vi "py-lvcomm.vi"() -> ()   [LabVIEW 2019]
uses:
  <vilib>/addons/zeromq/zmq_context.lvclass
  <vilib>/addons/zeromq/zmq_socket.lvclass
  <userlib>/LevyLab/Transport/Control Experiment/Control Experiment.lvclass
  <vilib>/addons/zeromq/socket_type.ctl
  <userlib>/LevyLab/Instrument Framework/Instrument Types/Cryostat/Instrument.Cryostat.lvclass
  <vilib>/addons/zeromq/zeromq.lvlib
  <userlib>/LevyLab/Lockin-Multichannel/Instrument.Lockin/Instrument.Lockin.lvclass
panel:
  out "Status":string
  out "Command":string
  in  "Exit":bool
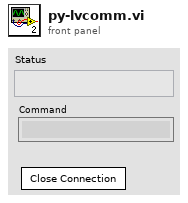
[diagram p1: front panel]
types:
  T1 = enum32{"Invalid", "Standard", "Closed", "Hidden", "Minimized", "Maximized"}
  T2 = enum32{"invalid app kind", "Development System", "Run Time System", "Student Edition", "Embedded LabVIEW", "Evaluation", "Custom"}
  T3 = typedef "zeromq.lvlib/socket_type.ctl" = enum8{"ZMQ_PAIR", "ZMQ_PUB", "ZMQ_SUB", "ZMQ_REQ", "ZMQ_REP", "ZMQ_DEALER", "ZMQ_ROUTER", "ZMQ_PULL", "ZMQ_PUSH", "ZMQ_XPUB", "ZMQ_XSUB", "ZMQ_STREAM", "ZMQ_SERVER", "ZMQ_CLIENT", "ZMQ_RADIO", "ZMQ_DISH", "ZMQ_GATHER", "ZMQ_SCATTER", "ZMQ_DGRAM"}
  T4 = cluster{"Core":cluster{"Current VI Reference":refnum<vi>, "Close Panel on Exit?":bool}, "ZMQ":cluster{"Context":refnum<class "zmq_context.lvclass">, "Socket":refnum<class "zmq_socket.lvclass">}, "C.E.":refnum<class "Control Experiment.lvclass">, "Command":cluster{"Command":string, "Args":string}}
  T5 = cluster{"Context":refnum<class "zmq_context.lvclass">, "Socket":refnum<class "zmq_socket.lvclass">}
  T6 = cluster{"Current VI Reference":refnum<vi>, "Close Panel on Exit?":bool}
  T7 = typedef "Control Experiment.lvclass/Instrument Classes--cluster.ctl" = cluster{"KH7008":refnum<class "Instrument.KH7008.lvclass">[], "Lockin":refnum<class "Instrument.Lockin.lvclass">, "Temperature":refnum<class "Instrument.Cryostat.lvclass">, "Magnet":refnum<class "Instrument.Cryostat.lvclass">, "Rotator":refnum<class "Instrument.Cryostat.lvclass">, "Level":refnum<class "Instrument.Cryostat.lvclass">, "Capacitance Bridge":refnum<class "Instrument.CBridge.lvclass">, "Delay Line":refnum<class "Instrument.DelayLine.lvclass">, "Strain Cell":refnum<class "Instrument.Strain.lvclass">, "VNA":refnum<class "Instrument.VNA.lvclass">, "Voltage Source":refnum<class "Instrument.VSource.lvclass">}
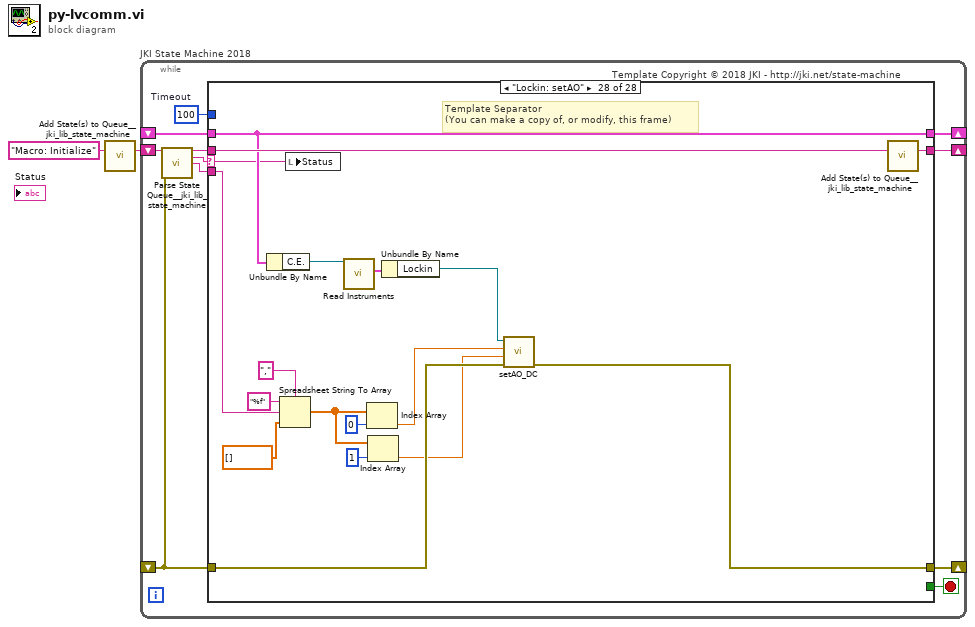
[diagram p0: block diagram]
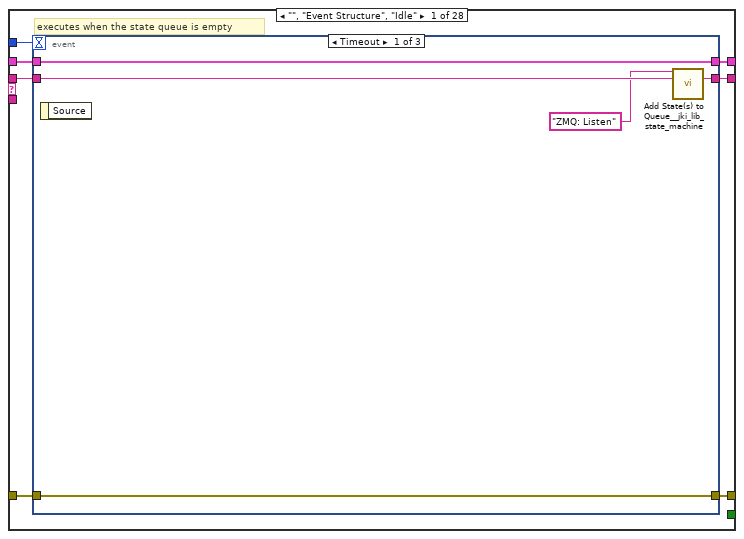
[diagram p2: hidden frame]
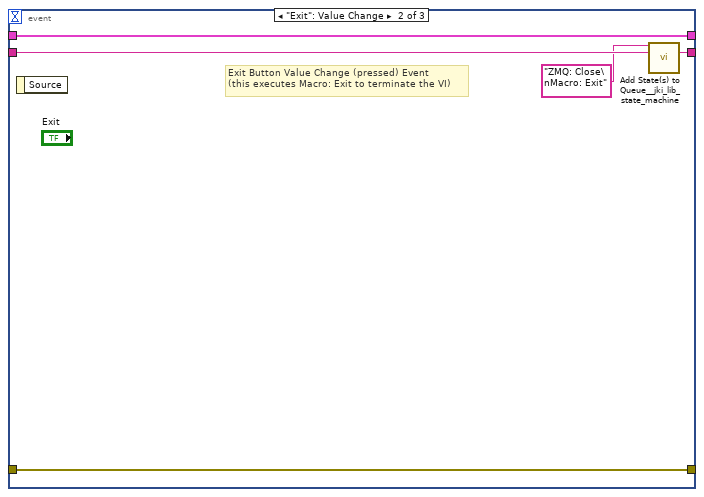
[diagram p3: hidden frame]
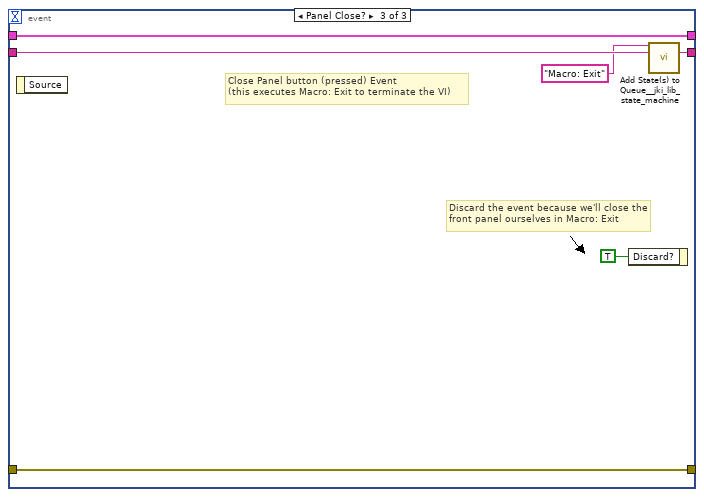
[diagram p4: hidden frame]
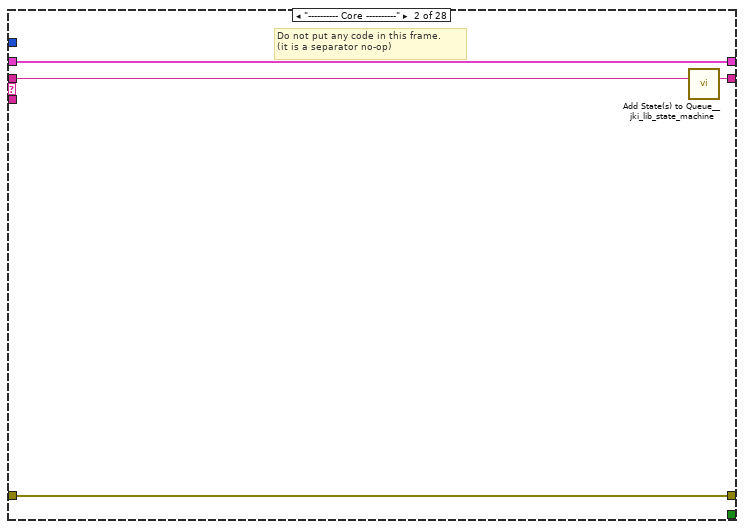
[diagram p5: hidden frame]
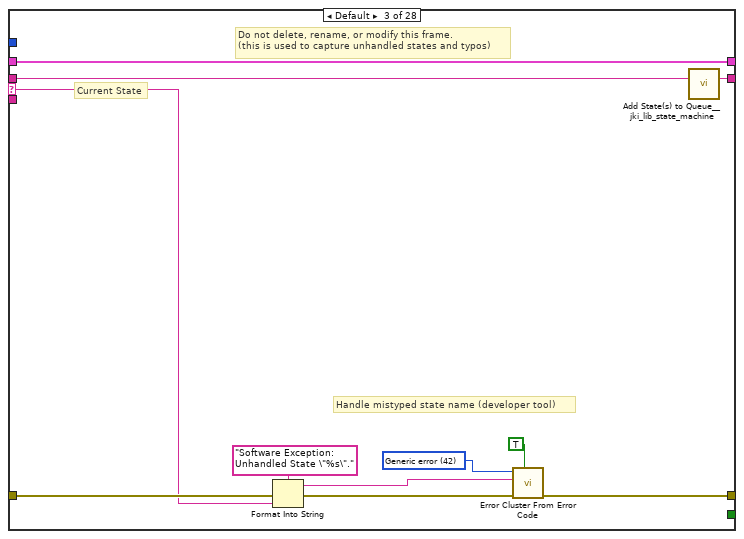
[diagram p6: hidden frame]
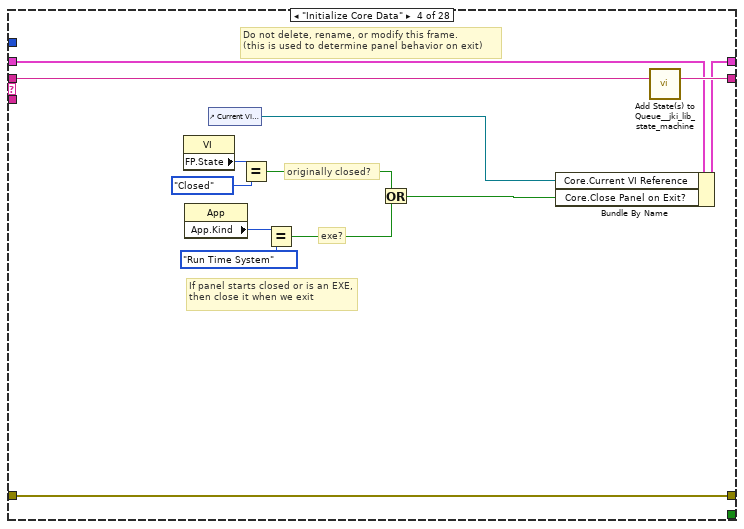
[diagram p7: hidden frame]
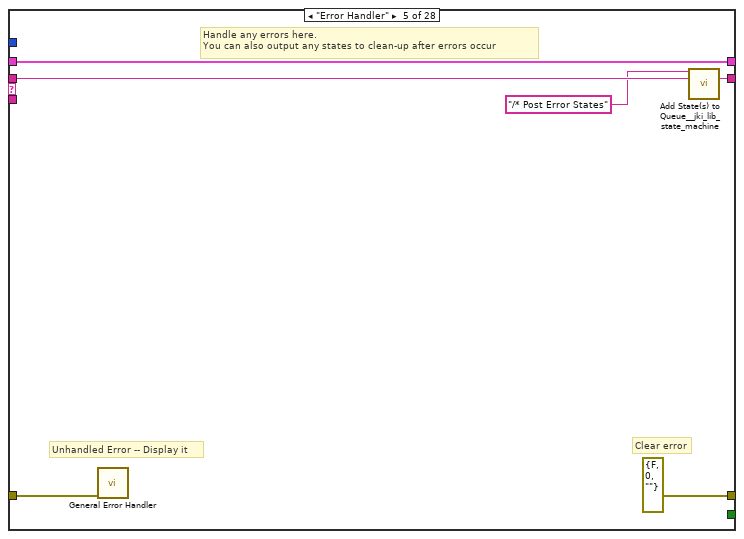
[diagram p8: hidden frame]
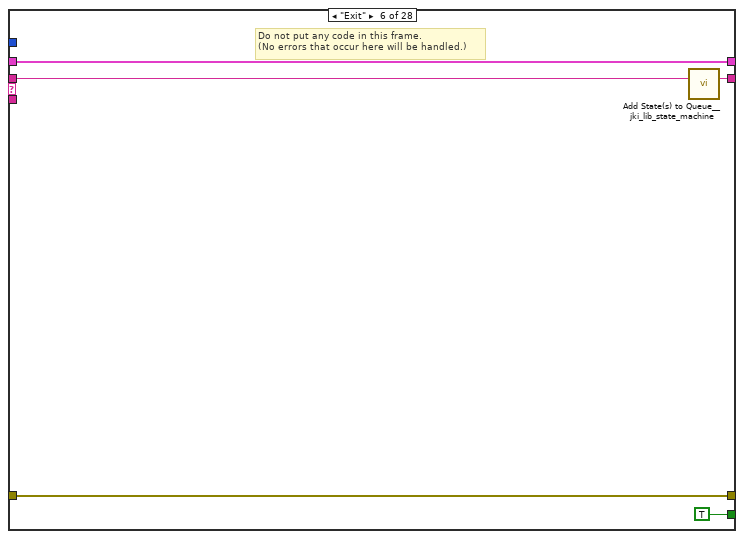
[diagram p9: hidden frame]
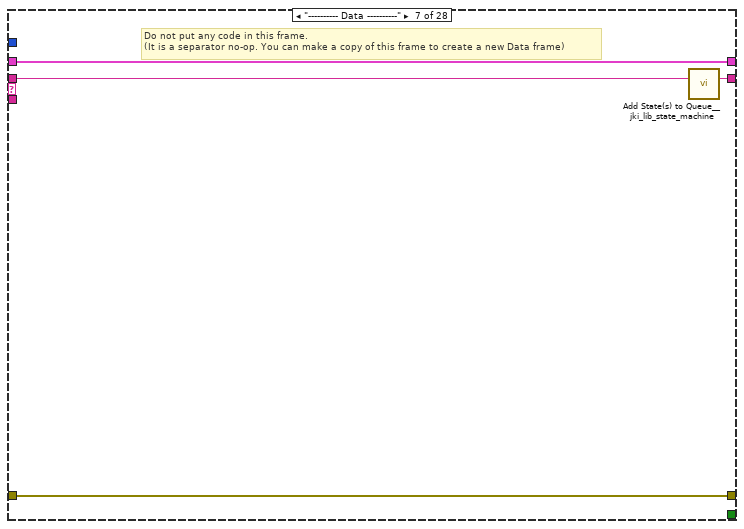
[diagram p10: hidden frame]
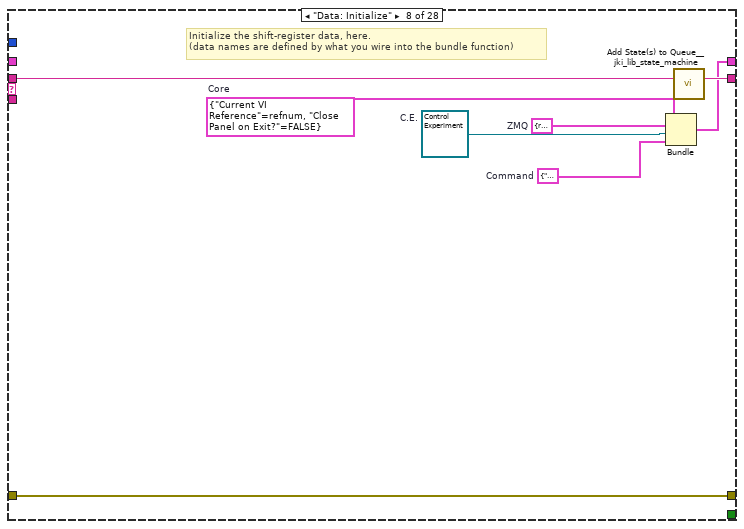
[diagram p11: hidden frame]
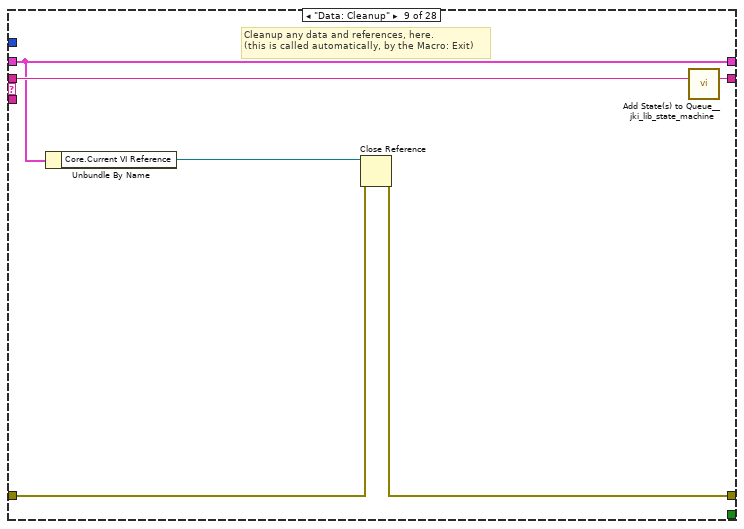
[diagram p12: hidden frame]
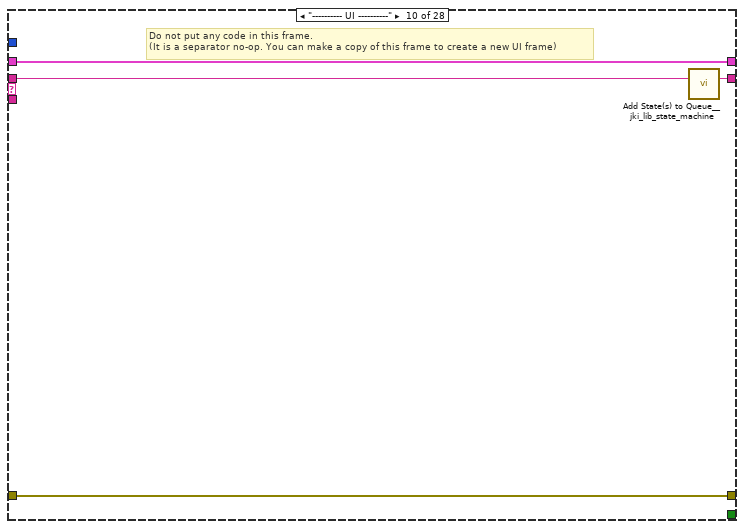
[diagram p13: hidden frame]
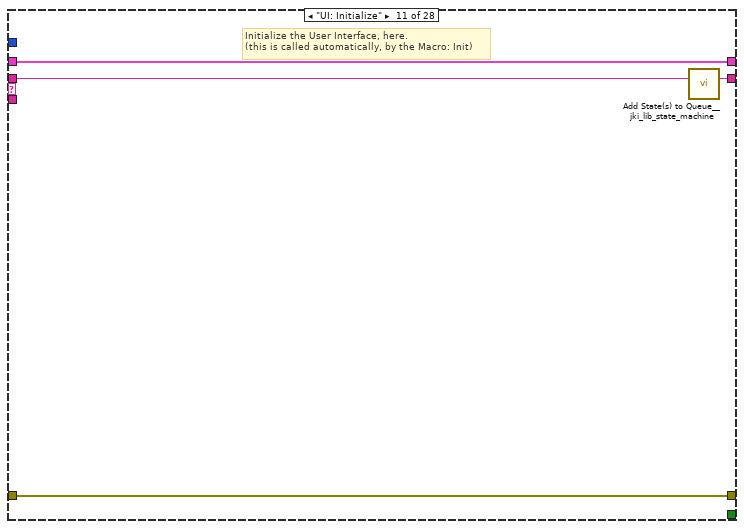
[diagram p14: hidden frame]
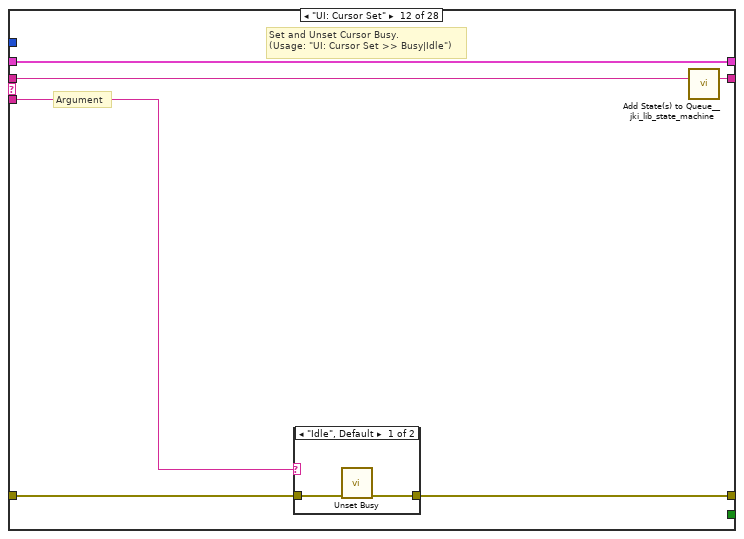
[diagram p15: hidden frame]
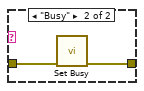
[diagram p16: hidden frame]
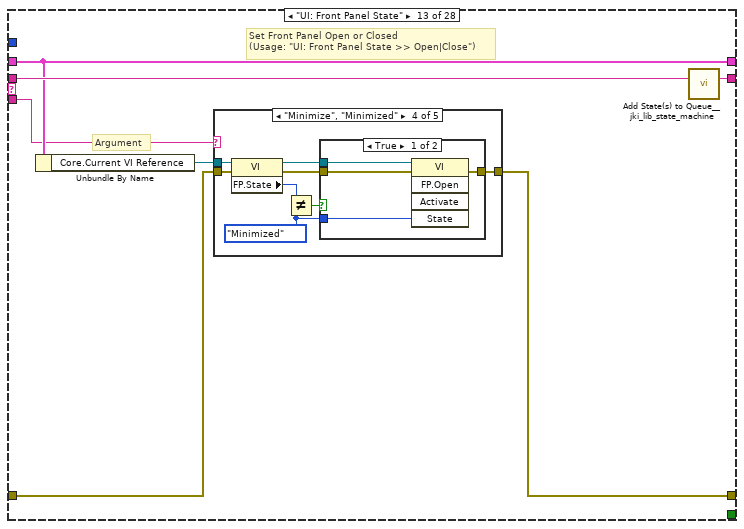
[diagram p17: hidden frame]
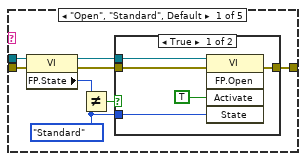
[diagram p18: hidden frame]
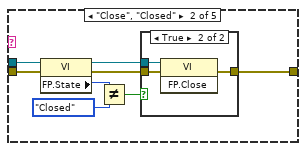
[diagram p20: hidden frame]
diagram:
  n1 = call <vilib>:"Add State(s) to Queue__jki_lib_state_machine.vi"("State(s) in (\"\")"="Macro: Initialize") -> ("States Out"=w2:string)  [unwired: 14 in]
  n2 = while "JKI State Machine 2018" {
    shift-right: [w6] -> _
    shift-left: _ -> [w5]
    shift-right: [w9] -> _
    shift-left: _ -> [w3]
    shift-right: [w8] -> _
    shift-left: w2 -> [w10]
    stop <- w7 stop-if-true
    w4 = 100  # Timeout
    # "Template Copyright © 2018 JKI - http://jki.net/state-machine"
    n3 = call <vilib>:"Parse State Queue__jki_lib_state_machine.vi"("State Queue"=w10, "Error In (no error)"=w3) -> ("Remaining States"=w12:string, "Current State"=w13:string, "Arguments"=w11:string)  [unwired: 11 in]
    n4 = case shown="\"Lockin: setAO\"" w13 {
      selector: w13 -> [_ _ w41 _ _ _ _ _ _ _ _ _ _ _ _ _ _ w207 w228 w245 _ _ _ _ w292 w311 _ w334]
      tunnel: w12 -> [w20 w40 w45 w64 w70 w75 w79 w87 w93 w97 w101 w107 w118 w187 w192 w202 w206 w221 w242 w250 w266 w270 w278 w282 w301 w320 w324 w342]
      tunnel: w11 -> [_ _ _ _ _ _ _ _ _ _ _ w102 w112 _ _ _ _ _ _ _ _ _ _ _ w291 w310 _ w327]
      tunnel: w5 -> [w18 w37 w43 w57 w67 w73 w76 _ w88 w94 w99 w105 w114 w184 w189 w199 w203 w211 w236 w246 w264 w267 w275 w279 w298 w317 w321 w338]
      tunnel: [w17 w38 w47 w61 errorcluster {"status"=FALSE, "code"=0, "source"=""} ("error out") w72 w77 w84 w89 w95 w98 w103 w115 w185 w190 w200 w204 w212 w233 w247 w259 w268 w273 w280 w294 w313 w322 w339] -> w9
      tunnel: w3 -> [w16 w38 w46 w61 w66 w72 w77 w84 w90 w95 w98 w104 w116 w185 w190 w200 w204 w216 w239 w247 w261 w268 w272 w280 w296 w315 w322 w340]
      tunnel: [w19 w39 w44 w63 w69 w74 w78 w86 w92 w96 w100 w106 w117 w186 w191 w201 w205 w220 w241 w249 w265 w269 w277 w281 w300 w319 w323 w341] -> w8
      tunnel: [_ _ _ _ _ TRUE _ _ _ _ _ _ _ _ _ _ _ _ _ _ _ _ _ _ _ _ _ _] -> w7
      tunnel: [w15 w37 w43 w62 w67 w73 w76 w85 w88 w94 w99 w105 w114 w184 w189 w199 w203 w210 w235 w246 w264 w267 w271 w279 w298 w317 w321 w338] -> w6
      tunnel: w4 -> [w14 _ _ _ _ _ _ _ _ _ _ _ _ _ _ _ _ _ _ _ _ _ _ _ _ _ _ _]
      frame "", "Event Structure", "Idle" {
        # "executes when the state queue is empty"
        n5 = event shown="[0] Timeout" {
          selector: _ -> [_ _ _]
          dyn-events: _ -> [_ _ _]
          timeout: w14 -> [_ _ _]
          tunnel: w20 -> [w25 w30 w36]
          tunnel: [w24 w29 w35] -> w19
          tunnel: w18 -> [w22 w27 w33]
          tunnel: [w23 w28 w34] -> w17
          tunnel: w16 -> [w23 w28 w34]
          tunnel: [w22 w27 w33] -> w15
          event Timeout {
            n6 = event-data() -> ()  [unwired: 1 in, 1 out]
            n7 = call <vilib>:"Add State(s) to Queue__jki_lib_state_machine.vi"("State(s) in Front (\"\")"="ZMQ: Listen" ("State(s) in Front (\"\")"), "State(s) in (\"\")"=w25) -> ("States Out"=w24:string)  [unwired: 13 in]
          }
          event "Exit": Value Change {
            # "Exit Button Value Change (pressed) Event\n(this executes Macro: Exit to terminate the VI)"
            n8 = event-data() -> ()  [unwired: 1 in, 1 out]
            n9 = call <vilib>:"Add State(s) to Queue__jki_lib_state_machine.vi"("State(s) in Front (\"\")"="ZMQ: Close\nMacro: Exit", "State(s) in (\"\")"=w30) -> ("States Out"=w29:string)  [unwired: 13 in]
          }
          event Panel Close? {
            # "Discard the event because we'll close the front panel ourselves in Macro: Exit"
            # "Close Panel button (pressed) Event\n(this executes Macro: Exit to terminate the VI)"
            n10 = event-data() -> ()  [unwired: 1 in, 1 out]
            n11 = event-data("Discard?"=TRUE) -> ()  [unwired: 1 in, 1 out]
            n12 = call <vilib>:"Add State(s) to Queue__jki_lib_state_machine.vi"("State(s) in Front (\"\")"="Macro: Exit", "State(s) in (\"\")"=w36) -> ("States Out"=w35:string)  [unwired: 13 in]
          }
        }
      }
      frame "---------- Core ----------" {
        # "Do not put any code in this frame.\n(it is a separator no-op)"
        n13 = call <vilib>:"Add State(s) to Queue__jki_lib_state_machine.vi"("State(s) in (\"\")"=w40) -> ("States Out"=w39:string)  [unwired: 14 in]
      }
      frame Default {
        w50 = 42 items=["No error", "Argument error", "Memory is full", "Out of zone", "End of file", "File already open", "Generic file I/O error", "File not found", "File permission error", "Disk is full", "Duplicate path", "Too many files open", "System feature not enabled", "Resource file not found", "Cannot add resource", "Resource not found", "Image not found", "Image memory error", "Pen does not exist", "Config type invalid", "Config token not found", "Config parse error", "Config memory error", "Bad external code format", "Bad external code offset", "External code not present", "Null window", "Destroy window error", "Null menu", "Print aborted", "Bad print record", "Print driver error", "Windows error during printing", "Memory error during printing", "Print dialog error", "Generic print error", "Invalid device refnum", "Device not found", "Device parameter error", "Device unit error", "Cannot open device", "Device call aborted", "Generic error", "Cancelled by user", "Object ID too low", "Object ID too high", "Object not in heap", "Unknown heap", "Unknown object (invalid DefProc)", "Unknown object (DefProc not in table)", "Message out of range", "Invalid (null) method", "Unknown message", "Manager call not supported", "Bad address", "Network operation in progress", "Network operation timed out", "Connection is busy", "Network attribute not supported", "Network error", "Address in use", "System out of memory", "Connection aborted", "Connection refused", "Not connected", "Already connected", "Connection closed", "Initialization error (interapplication manager)", "Bad occurrence", "Wait on unbound occurrence handler", "Occurrence queue overflow", "Datalog type conflict", "Unused", "Unrecognized type (interapplication manager)", "Memory corrupt", "Failed to make temporary DLL", "Old CIN version", "Drag socket not found", "Failed to load drop-object", "Failed to register OLE object", "Failed to release OLE object", "Format specifier type mismatch", "Unknown format specifier", "Too few format specifiers", "Too many format specifiers", "Scan failed", "Newer CIN version", "Error converting to variant", "Runtime menu error", "Password tampered", "Variant attribute not found", "Incompatible variant data type", "Event data is not available", "Event Store is not present", "Occurrence is not found", "Event Queue is not created", "Event info is not available", "Refnum passed is NULL", "Error retrieving Class GUID", "Error retrieving CoClass GUID", "Error retrieving TypeLib GUID.", "Bad built application magic bytes.", "Specific driver is different from the specific driver associated with the Logical Name.", "There is no session opened to the class driver.", "Max Error", "MAX - Error with config objects", "MAX - Error loading configuration", "MAX - Group not supported"]
        # "Current State"
        # "Do not delete, rename, or modify this frame.\n(this is used to capture unhandled states and typos)"
        # "Handle mistyped state name (developer tool)"
        n14 = Format Into String(format string="Software Exception: Unhandled State \"%s\"." ("message"), error in=w46, w41) -> (resulting string=w49:string, error out=w48:errorcluster)  [unwired: 1 in]
        n15 = call <vilib>:"Error Cluster From Error Code.vi"("show call chain? (False)"=TRUE, "error in (no error)"=w48, "error message (\"\")"=w49, "error code (0)"=w50) -> ("error out"=w47:errorcluster)  [unwired: 5 in]
        n16 = call <vilib>:"Add State(s) to Queue__jki_lib_state_machine.vi"("State(s) in (\"\")"=w45) -> ("States Out"=w44:string)  [unwired: 14 in]
      }
      frame "Initialize Core Data" {
        # "Do not delete, rename, or modify this frame.\n(this is used to determine panel behavior on exit)"
        # "originally closed?"
        # "exe?"
        # "If panel starts closed or is an EXE, then close it when we exit"
        n17 = property class="VI"() -> ("FP.State"=w54:T1)  [unwired: 2 in, 2 out]
        n18 = property class="App"() -> ("App.Kind"=w60:T2)  [unwired: 2 in, 2 out]
        n19 = control-ref of="Current VI Reference"() -> (w55:refnum<vi>)
        n20 = Equal?(x=w54, y=T1."Closed" ("Front Panel Window:State")) -> (x = y?=w52:bool)
        n21 = Equal?(x=w60, y=T2."Run Time System" ("Application:Kind")) -> (x = y?=w58:bool)
        n22 = Or(x=w52, y=w58) -> (x .or. y?=w56:bool)
        n23 = Bundle By Name(cluster=w57, "Core.Current VI Reference"=w55, "Core.Close Panel on Exit?"=w56) -> (w62:T4)
        n24 = call <vilib>:"Add State(s) to Queue__jki_lib_state_machine.vi"("State(s) in (\"\")"=w64) -> ("States Out"=w63:string)  [unwired: 14 in]
      }
      frame "Error Handler" {
        # "Unhandled Error -- Display it"
        # "Handle any errors here.\nYou can also output any states to clean-up after errors occur"
        # "Clear error"
        n25 = call <vilib>:"General Error Handler.vi"("error in (no error)"=w66) -> ()  [unwired: 10 in, 5 out]
        n26 = call <vilib>:"Add State(s) to Queue__jki_lib_state_machine.vi"("State(s) in Front (\"\")"="/* Post Error States", "State(s) in (\"\")"=w70) -> ("States Out"=w69:string)  [unwired: 13 in]
      }
      frame "Exit" {
        # "Do not put any code in this frame.\n(No errors that occur here will be handled.)"
        n27 = call <vilib>:"Add State(s) to Queue__jki_lib_state_machine.vi"("State(s) in (\"\")"=w75) -> ("States Out"=w74:string)  [unwired: 14 in]
      }
      frame "---------- Data ----------" {
        # "Do not put any code in this frame.\n(It is a separator no-op. You can make a copy of this frame to create a new Data frame)"
        n28 = call <vilib>:"Add State(s) to Queue__jki_lib_state_machine.vi"("State(s) in (\"\")"=w79) -> ("States Out"=w78:string)  [unwired: 14 in]
      }
      frame "Data: Initialize" {
        w80 = cluster{"Command":string, "Args":string} {"Command"="", "Args"=""}  # Command
        w81 = refnum<class "Control Experiment.lvclass"> refnum  # C.E.
        w82 = T5 {"Context"=refnum, "Socket"=refnum}  # ZMQ
        w83 = T6 {"Current VI Reference"=refnum, "Close Panel on Exit?"=FALSE}  # Core
        # "Initialize the shift-register data, here.\n(data names are defined by what you wire into the bundle function)"
        n29 = Bundle("Core"=w83, "ZMQ"=w82, "C.E."=w81, "Command"=w80) -> (w85:T4)  [unwired: 1 in]
        n30 = call <vilib>:"Add State(s) to Queue__jki_lib_state_machine.vi"("State(s) in (\"\")"=w87) -> ("States Out"=w86:string)  [unwired: 14 in]
      }
      frame "Data: Cleanup" {
        # "Cleanup any data and references, here.\n(this is called automatically, by the Macro: Exit)"
        n31 = Unbundle By Name(w88) -> ("Core.Current VI Reference"=w91:refnum<vi>)
        n32 = Close Reference(reference=w91, error in (no error)=w90) -> (error out=w89:errorcluster)
        n33 = call <vilib>:"Add State(s) to Queue__jki_lib_state_machine.vi"("State(s) in (\"\")"=w93) -> ("States Out"=w92:string)  [unwired: 14 in]
      }
      frame "---------- UI ----------" {
        # "Do not put any code in this frame.\n(It is a separator no-op. You can make a copy of this frame to create a new UI frame)"
        n34 = call <vilib>:"Add State(s) to Queue__jki_lib_state_machine.vi"("State(s) in (\"\")"=w97) -> ("States Out"=w96:string)  [unwired: 14 in]
      }
      frame "UI: Initialize" {
        # "Initialize the User Interface, here.\n(this is called automatically, by the Macro: Init)"
        n35 = call <vilib>:"Add State(s) to Queue__jki_lib_state_machine.vi"("State(s) in (\"\")"=w101) -> ("States Out"=w100:string)  [unwired: 14 in]
      }
      frame "UI: Cursor Set" {
        # "Argument"
        # "Set and Unset Cursor Busy.\n(Usage: \"UI: Cursor Set >> Busy|Idle\")"
        n36 = case shown="\"Idle\", Default" w102 {
          tunnel: w104 -> [w109 w111]
          tunnel: [w108 w110] -> w103
          frame "Idle", Default {
            n37 = call <vilib>:"Unset Busy.vi"("error in (no error)"=w109) -> ("error out"=w108:errorcluster)  [unwired: 10 in]
          }
          frame "Busy" {
            n38 = call <vilib>:"Set Busy.vi"("error in (no error)"=w111) -> ("error out"=w110:errorcluster)  [unwired: 9 in, 1 out]
          }
        }
        n39 = call <vilib>:"Add State(s) to Queue__jki_lib_state_machine.vi"("State(s) in (\"\")"=w107) -> ("States Out"=w106:string)  [unwired: 14 in]
      }
      frame "UI: Front Panel State" {
        # "Argument"
        # "Set Front Panel Open or Closed\n(Usage: \"UI: Front Panel State >> Open|Close\")"
        n40 = Unbundle By Name(w114) -> ("Core.Current VI Reference"=w113:refnum<vi>)
        n41 = case shown="\"Minimize\", \"Minimized\"" w112 {
          tunnel: w116 -> [w124 w139 w150 w163 w176]
          tunnel: [w126 w140 w152 w165 w178] -> w115
          tunnel: w113 -> [w125 w137 w151 w164 w177]
          frame "Open", "Standard", Default {
            w119 = T1."Standard" ("State")
            n42 = property class="VI"(reference=w125, error in=w124) -> (reference out=w122:refnum<vi>, error out=w123:errorcluster, "FP.State"=w121:T1)
            n43 = Not Equal?(x=w121, y=w119) -> (x != y?=w120:bool)
            n44 = case shown="True" w120 {
              tunnel: [w130 w132] -> w126
              tunnel: w123 -> [w129 w132]
              tunnel: w122 -> [w128 _]
              tunnel: w119 -> [w127 _]
              frame True {
                n45 = invoke class="VI" method="FP.Open"(reference=w128, error in=w129, "Activate"=TRUE, "State"=w127) -> (error out=w130:errorcluster)  [unwired: 1 in, 4 out]
              }
              frame False {
              }
            }
          }
          frame "Close", "Closed" {
            n46 = property class="VI"(reference=w137, error in=w139) -> (reference out=w136:refnum<vi>, error out=w138:errorcluster, "FP.State"=w134:T1)
            n47 = Not Equal?(x=w134, y=T1."Closed" ("Front Panel Window:State")) -> (x != y?=w133:bool)
            n48 = case shown="True" w133 {
              tunnel: [w141 w144] -> w140
              tunnel: w138 -> [w141 w143]
              tunnel: w136 -> [_ w142]
              frame False {
              }
              frame True {
                n49 = invoke class="VI" method="FP.Close"(reference=w142, error in=w143) -> (error out=w144:errorcluster)  [unwired: 1 in, 2 out]
              }
            }
          }
          frame "Hidden", "Hide" {
            w145 = T1."Hidden" ("State")
            n50 = property class="VI"(reference=w151, error in=w150) -> (reference out=w148:refnum<vi>, error out=w149:errorcluster, "FP.State"=w147:T1)
            n51 = Not Equal?(x=w147, y=w145) -> (x != y?=w146:bool)
            n52 = case shown="True" w146 {
              tunnel: [w156 w157] -> w152
              tunnel: w149 -> [w155 w157]
              tunnel: w148 -> [w154 _]
              tunnel: w145 -> [w153 _]
              frame True {
                n53 = invoke class="VI" method="FP.Open"(reference=w154, error in=w155, "State"=w153) -> (error out=w156:errorcluster)  [unwired: 2 in, 4 out]
              }
              frame False {
              }
            }
          }
          frame "Minimize", "Minimized" {
            w158 = T1."Minimized" ("State")
            n54 = property class="VI"(reference=w164, error in=w163) -> (reference out=w161:refnum<vi>, error out=w162:errorcluster, "FP.State"=w160:T1)
            n55 = Not Equal?(x=w160, y=w158) -> (x != y?=w159:bool)
            n56 = case shown="True" w159 {
              tunnel: [w169 w170] -> w165
              tunnel: w162 -> [w168 w170]
              tunnel: w161 -> [w167 _]
              tunnel: w158 -> [w166 _]
              frame True {
                n57 = invoke class="VI" method="FP.Open"(reference=w167, error in=w168, "State"=w166) -> (error out=w169:errorcluster)  [unwired: 2 in, 4 out]
              }
              frame False {
              }
            }
          }
          frame "Maximize", "Maximized" {
            w171 = T1."Maximized" ("State")
            n58 = property class="VI"(reference=w177, error in=w176) -> (reference out=w174:refnum<vi>, error out=w175:errorcluster, "FP.State"=w173:T1)
            n59 = Not Equal?(x=w173, y=w171) -> (x != y?=w172:bool)
            n60 = case shown="True" w172 {
              tunnel: [w182 w183] -> w178
              tunnel: w175 -> [w181 w183]
              tunnel: w174 -> [w180 _]
              tunnel: w171 -> [w179 _]
              frame True {
                n61 = invoke class="VI" method="FP.Open"(reference=w180, error in=w181, "State"=w179) -> (error out=w182:errorcluster)  [unwired: 2 in, 4 out]
              }
              frame False {
              }
            }
          }
        }
        n62 = call <vilib>:"Add State(s) to Queue__jki_lib_state_machine.vi"("State(s) in (\"\")"=w118) -> ("States Out"=w117:string)  [unwired: 14 in]
      }
      frame "---------- Macro ----------" {
        # "Do not put any code in this frame.\n(It is a separator no-op. You can make a copy of this frame to create a new Macro frame)"
        n63 = call <vilib>:"Add State(s) to Queue__jki_lib_state_machine.vi"("State(s) in (\"\")"=w187) -> ("States Out"=w186:string)  [unwired: 14 in]
      }
      frame "Macro: Initialize" {
        w188 = "Data: Initialize\nInitialize Core Data\nUI: Initialize\nUI: Front Panel State >> Open\nCE: Init\nZMQ: Init"  # Data: Initialize Initialize Core Data UI: Initialize UI: Front Panel State >> Open CE: Init ZMQ: Init
        # "Initialization Macro\n(This is called once, when the VI starts)"
        n64 = call <vilib>:"Add State(s) to Queue__jki_lib_state_machine.vi"("State(s) in Front (\"\")"=w188, "State(s) in (\"\")"=w192) -> ("States Out"=w191:string)  [unwired: 13 in]
      }
      frame "Macro: Exit" {
        # "Exit Macro\n(This is called once, when the VI exits)"
        n65 = Unbundle By Name(w199) -> ("Core.Close Panel on Exit?"=w198:bool)
        n66 = Select(t="UI: Front Panel State >> Close", s=w198, f="") -> (s? t:f=w195:string)
        n67 = call <vilib>:"Add State(s) to Queue__jki_lib_state_machine.vi"("State(s) in (\"\")"=w195, "State(s) at Back (\"\")"="Data: Cleanup\nExit") -> ("States Out"=w193:string)  [unwired: 13 in]
        n68 = call <vilib>:"Add State(s) to Queue__jki_lib_state_machine.vi"("State(s) in Front (\"\")"=w193, "State(s) in (\"\")"=w202) -> ("States Out"=w201:string)  [unwired: 13 in]
      }
      frame "---------- ZMQ ----------" {
        # "Template Separator\n(You can make a copy of, or modify, this frame)"
        n69 = call <vilib>:"Add State(s) to Queue__jki_lib_state_machine.vi"("State(s) in (\"\")"=w206) -> ("States Out"=w205:string)  [unwired: 14 in]
      }
      frame "ZMQ: Init" {
        n70 = local write "Status"(w207) -> ()
        n71 = call <vilib>:"zmq_ctx_create.vi"("error in"=w216) -> ("error out"=w215:errorcluster, "context out"=w219:refnum<class "zmq_context.lvclass">)  [unwired: 3 in]
        n72 = call <vilib>:"zmq_socket.vi"("error in"=w215, "socket type"=socket_type."ZMQ_REP", "context in"=w219) -> ("error out"=w213:errorcluster, "socket out"=w217:refnum<class "zmq_socket.lvclass">, "context out"=w209:refnum<class "zmq_context.lvclass">)  [unwired: 2 in]
        n73 = call <vilib>:"zmq_bind.vi"("error in"=w213, "endpoint"="tcp://*:15555", "socket in"=w217) -> ("error out"=w212:errorcluster, "socket out"=w208:refnum<class "zmq_socket.lvclass">)  [unwired: 1 in]
        n74 = Bundle By Name(cluster=w211, "ZMQ.Context"=w209, "ZMQ.Socket"=w208) -> (w210:T4)
        n75 = call <vilib>:"Add State(s) to Queue__jki_lib_state_machine.vi"("State(s) in (\"\")"=w221) -> ("States Out"=w220:string)  [unwired: 14 in]
      }
      frame "ZMQ: Listen" {
        # "Your code here.\n(You can make a copy of, or modify, this frame)"
        n76 = Unbundle By Name(w236) -> ("ZMQ.Socket"=w240:refnum<class "zmq_socket.lvclass">)
        n77 = local write "Status"(w228) -> ()
        n78 = call <vilib>:"zmq_recv.vi"("error in"=w239, "socket in"=w240) -> ("error out"=w237:errorcluster, "data"=w225:string, "socket out"=w238:refnum<class "zmq_socket.lvclass">)  [unwired: 3 in, 2 out]
        "Command" <- w225
        n79 = Format Into String(format string="Message Received: %s", w225) -> (resulting string=w231:string)  [unwired: 2 in, 1 out]
        n80 = call <vilib>:"zmq_send.vi"("error in"=w237, "data"=w231, "socket in"=w238) -> ("error out"=w233:errorcluster, "socket out"=w234:refnum<class "zmq_socket.lvclass">)  [unwired: 4 in]
        n81 = Match Pattern(string=w225, regular expression=":") -> (before substring=w223:string, after substring=w222:string)  [unwired: 1 in, 2 out]
        n82 = Empty String/Path?(string/path=w225) -> (empty?=w230:bool)
        n83 = Bundle By Name(cluster=w236, "ZMQ.Socket"=w234, "Command.Command"=w223, "Command.Args"=w222) -> (w235:T4)
        n84 = Select(t="", s=w230, f="ZMQ: Process") -> (s? t:f=w229:string)
        n85 = call <vilib>:"Add State(s) to Queue__jki_lib_state_machine.vi"("State(s) in Front (\"\")"=w229, "State(s) in (\"\")"=w242) -> ("States Out"=w241:string)  [unwired: 13 in]
      }
      frame "ZMQ: Process" {
        # "Your code here.\n(You can make a copy of, or modify, this frame)"
        n86 = Unbundle By Name(w246) -> ("Command.Command"=w244:string, "Command.Args"=w243:string)
        n87 = local write "Status"(w245) -> ()
        n88 = case shown="\"set_temp\"" w244 {
          tunnel: ["" ("State(s) in Front (\"\")") "" ("State(s) in Front (\"\")") w254 w257] -> w248
          tunnel: w243 -> [_ _ w253 w256]
          frame "set_field" {
          }
          frame Default {
          }
          frame "set_temp" {
            n89 = Format Into String(format string="PPMS: Set Temp >> %s ", w253) -> (resulting string=w254:string)  [unwired: 2 in, 1 out]
          }
          frame "set_AO" {
            n90 = Format Into String(format string="Lockin: setAO >> %s ", w256) -> (resulting string=w257:string)  [unwired: 2 in, 1 out]
          }
        }
        n91 = call <vilib>:"Add State(s) to Queue__jki_lib_state_machine.vi"("State(s) in Front (\"\")"=w248, "State(s) in (\"\")"=w250) -> ("States Out"=w249:string)  [unwired: 13 in]
      }
      frame "ZMQ: Close" {
        # "Your code here.\n(You can make a copy of, or modify, this frame)"
        n92 = Unbundle By Name(w264) -> ("ZMQ.Context"=w262:refnum<class "zmq_context.lvclass">, "ZMQ.Socket"=w263:refnum<class "zmq_socket.lvclass">)
        n93 = call <vilib>:"zmq_close.vi"("error in"=w261, "socket"=w263) -> ("error out"=w260:errorcluster)  [unwired: 3 in]
        n94 = call <vilib>:"zmq_ctx_destroy.vi"("error in"=w260, "context in"=w262) -> ("error out"=w259:errorcluster)  [unwired: 3 in]
        n95 = call <vilib>:"Add State(s) to Queue__jki_lib_state_machine.vi"("State(s) in (\"\")"=w266) -> ("States Out"=w265:string)  [unwired: 14 in]
      }
      frame "---------- CE ----------" {
        # "Template Separator\n(You can make a copy of, or modify, this frame)"
        n96 = call <vilib>:"Add State(s) to Queue__jki_lib_state_machine.vi"("State(s) in (\"\")"=w270) -> ("States Out"=w269:string)  [unwired: 14 in]
      }
      frame "CE: Init" {
        # "Template Separator\n(You can make a copy of, or modify, this frame)"
        n97 = call <userlib>:"Control Experiment FGV.vi"("Function"=enum16{"read", "write"}."read", "error in (no error)"=w272) -> ("error out"=w273:errorcluster, "Control Experiment.lvclass out"=w274:refnum<class "Control Experiment.lvclass">)  [unwired: 8 in]
        n98 = Bundle By Name(cluster=w275, "C.E."=w274) -> (w271:T4)
        n99 = call <vilib>:"Add State(s) to Queue__jki_lib_state_machine.vi"("State(s) in (\"\")"=w278) -> ("States Out"=w277:string)  [unwired: 14 in]
      }
      frame "---------- PPMS ----------" {
        # "Template Separator\n(You can make a copy of, or modify, this frame)"
        n100 = call <vilib>:"Add State(s) to Queue__jki_lib_state_machine.vi"("State(s) in (\"\")"=w282) -> ("States Out"=w281:string)  [unwired: 14 in]
      }
      frame "PPMS: Set Temp" {
        # "Template Separator\n(You can make a copy of, or modify, this frame)"
        n101 = Spreadsheet String To Array(delimiter (Tab)=",", format string="%f", spreadsheet string=w291, array type (2D Dbl)=dbl[] []) -> (array=w284:dbl[])
        n102 = local write "Status"(w292) -> ()
        n103 = Unbundle By Name(w298) -> ("C.E."=w297:refnum<class "Control Experiment.lvclass">)
        n104 = Index Array(array=w284, index=0) -> (element=w287:dbl)
        n105 = Index Array(array=w284, index=1) -> (element=w283:dbl)
        n106 = call <userlib>:"Read Instruments.vi"("error in (no error)"=w296, "Control Experiment in"=w297) -> ("error out"=w295:errorcluster, "Instruments"=w299:T7)  [unwired: 7 in, 1 out]
        n107 = Unbundle By Name(w299) -> ("Temperature"=w293:refnum<class "Instrument.Cryostat.lvclass">)
        n108 = call-dynamic "Set Temperature.vi"("error in (no error)"=w295, "Rate (K/min)"=w283, "Temperature (K)"=w287, "Instrument.Cryostat in"=w293) -> ("error out"=w294:errorcluster)  [unwired: 6 in, 1 out]
        n109 = call <vilib>:"Add State(s) to Queue__jki_lib_state_machine.vi"("State(s) in (\"\")"=w301) -> ("States Out"=w300:string)  [unwired: 14 in]
      }
      frame "PPMS: Set Field" {
        # "Template Separator\n(You can make a copy of, or modify, this frame)"
        n110 = Spreadsheet String To Array(delimiter (Tab)=",", format string="%f", spreadsheet string=w310, array type (2D Dbl)=dbl[] []) -> (array=w303:dbl[])
        n111 = local write "Status"(w311) -> ()
        n112 = Unbundle By Name(w317) -> ("C.E."=w316:refnum<class "Control Experiment.lvclass">)
        n113 = Index Array(array=w303, index=0) -> (element=w306:dbl)
        n114 = Index Array(array=w303, index=1) -> (element=w302:dbl)
        n115 = call <userlib>:"Read Instruments.vi"("error in (no error)"=w315, "Control Experiment in"=w316) -> ("error out"=w314:errorcluster, "Instruments"=w318:T7)  [unwired: 7 in, 1 out]
        n116 = Unbundle By Name(w318) -> ("Magnet"=w312:refnum<class "Instrument.Cryostat.lvclass">)
        n117 = call-dynamic "Set Temperature.vi"("error in (no error)"=w314, "Rate (K/min)"=w302, "Temperature (K)"=w306, "Instrument.Cryostat in"=w312) -> ("error out"=w313:errorcluster)  [unwired: 6 in, 1 out]
        n118 = call <vilib>:"Add State(s) to Queue__jki_lib_state_machine.vi"("State(s) in (\"\")"=w320) -> ("States Out"=w319:string)  [unwired: 14 in]
      }
      frame "---------- Lockin ----------" {
        # "Template Separator\n(You can make a copy of, or modify, this frame)"
        n119 = call <vilib>:"Add State(s) to Queue__jki_lib_state_machine.vi"("State(s) in (\"\")"=w324) -> ("States Out"=w323:string)  [unwired: 14 in]
      }
      frame "Lockin: setAO" {
        # "Template Separator\n(You can make a copy of, or modify, this frame)"
        n120 = Unbundle By Name(w338) -> ("C.E."=w337:refnum<class "Control Experiment.lvclass">)
        n121 = Spreadsheet String To Array(delimiter (Tab)=",", format string="%f", spreadsheet string=w327, array type (2D Dbl)=dbl[] []) -> (array=w328:dbl[])
        n122 = local write "Status"(w334) -> ()
        n123 = call <userlib>:"Read Instruments.vi"("Control Experiment in"=w337) -> ("Instruments"=w336:T7)  [unwired: 8 in, 2 out]
        n124 = Index Array(array=w328, index=0) -> (element=w326:dbl)
        n125 = Index Array(array=w328, index=1) -> (element=w325:dbl)
        n126 = Unbundle By Name(w336) -> ("Lockin"=w335:refnum<class "Instrument.Lockin.lvclass">)
        n127 = call <userlib>:"setAO_DC.vi"("error in (no error)"=w340, "DC (V)"=w325, "AO Channel"=w326, "Instrument.Lockin in"=w335) -> ("error out"=w339:errorcluster)  [unwired: 6 in, 1 out]
        n128 = call <vilib>:"Add State(s) to Queue__jki_lib_state_machine.vi"("State(s) in (\"\")"=w342) -> ("States Out"=w341:string)  [unwired: 14 in]
      }
    }
  }
